vi "String Subset.vi"() -> ()   [LabVIEW 2016]
panel:
  in  "Length":dbl
  in  "Offset":dbl
  out "String 2":string
  in  "String":string
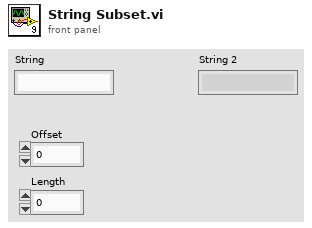
[diagram p1: front panel]
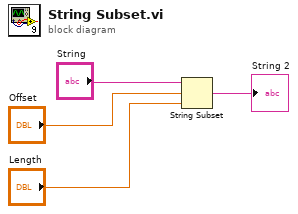
[diagram p0: block diagram]
diagram:
  n1 = String Subset(string="String", offset (0)="Offset", length (rest)="Length") -> (substring=→"String 2":string)
